vi "calcNewOutputs.vi"(8 "error in (no error)":errorcluster, 11 "Model in":refnum<class "Model.lvclass">) -> (0 "error out":errorcluster, 3 "Model out":refnum<class "Model.lvclass">)   [LabVIEW 2012, in "Model.lvclass"]
uses:
  Model.lvclass
  Model.lvclass/Model.ctl
  StreamingDataAlgorithm/StreamingDataAlgorithm.lvclass
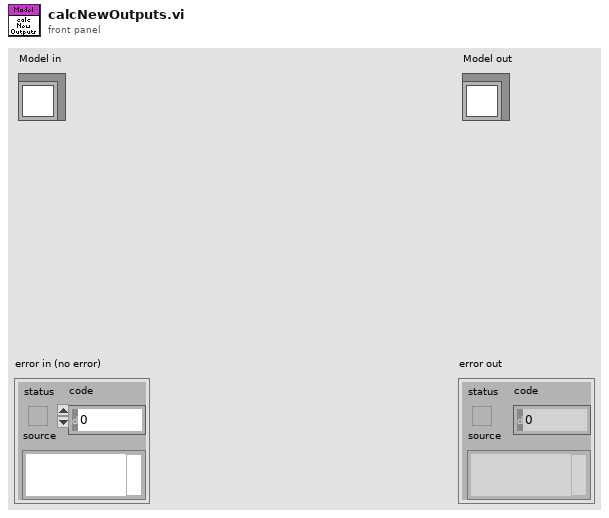
[diagram p1: front panel]
types:
  T1 = typedef "ILCCommon.lvlib/ILCTypedefs.lvlib/OutputData.ctl" = cluster{"Step & Direction":i16, "Blower RPM":u8, "PWM (SSR)":u8, "Ch1":u16, "Ch2":u16, "Ch3":u16, "Ch4":u16}
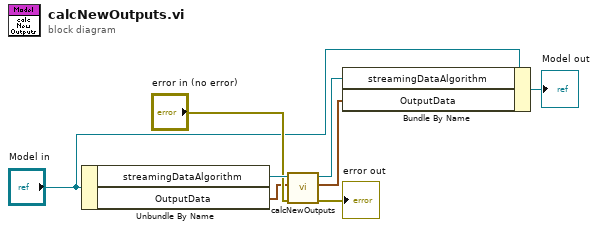
[diagram p0: block diagram]
diagram:
  n1 = Unbundle By Name("Model in") -> ("streamingDataAlgorithm"=w8:refnum<class "StreamingDataAlgorithm.lvclass">, "OutputData"=w1:T1)
  n2 = call-dynamic "calcNewOutputs.vi"("error in (no error)"="error in (no error)", "outputData"=w1, "StreamingDataAlgorithm in"=w8) -> ("error out"=→"error out":errorcluster, "outputData 2"=w2:T1, "StreamingDataAlgorithm out"=w5:refnum<class "StreamingDataAlgorithm.lvclass">)  [unwired: 6 in]
  n3 = Bundle By Name(cluster="Model in", "streamingDataAlgorithm"=w5, "OutputData"=w2) -> (→"Model out":refnum<class "Model.lvclass">)
